vi "PlotData Loop.vi"(8 "error in":errorcluster, 9 "IBM OptoElectroMechanics Configuration":T1={"Parameter Analizer"={"Parameter Analyzer VISA Session"="COM1", "Sweeping Time Parameters"={"Integration Time"=0, "Short Integration Time (s)"=1.0, "Long Integration Time (s)"=0.0, "Wait Time Parameter"=1.0}, "Acquisition Mode"=enum."Sweeping Mode", "Status Polling Time (ms)"=0, "Comment"="Test VI", "SMU 1 - Sweeping"={"Start / Offset"=0.0, "Stop / Ratio"=1.0, "Step \n(linear only)"=0.01, "Compliance"=0.1, "Power \nCompliance"=0.0, "Mode"=0, "Function"=0, "Sweep Mode"=FALSE}, "SMU 2 - Sweeping"={"Start / Offset"=0.0, "Stop / Ratio"=1.0, "Step \n(linear only)"=0.01, "Compliance"=0.1, "Power \nCompliance"=0.0, "Mode"=0, "Function"=0, "Sweep Mode"=FALSE}, "SMU 3 - Sweeping"={"Start / Offset"=0.0, "Stop / Ratio"=1.0, "Step \n(linear only)"=0.01, "Compliance"=0.1, "Power \nCompliance"=0.0, "Mode"=0, "Function"=0, "Sweep Mode"=FALSE}, "SMU 4 - Sweeping"={"Start / Offset"=0.0, "Stop / Ratio"=1.0, "Step \n(linear only)"=0.01, "Compliance"=0.1, "Power \nCompliance"=0.0, "Mode"=0, "Function"=0, "Sweep Mode"=FALSE}, "Sweep Spacing"=0, "Range"=0, "SMU1 - Sampling"={"Source"=10.0, "Compliance"=1e-05, "Mode"=0, "Function"=FALSE}, "SMU2 - Sampling"={"Source"=1.0, "Compliance"=1.0, "Mode"=0, "Function"=FALSE}, "SMU3 - Sampling"={"Source"=10.0, "Compliance"=1e-05, "Mode"=0, "Function"=FALSE}, "SMU4 - Sampling"={"Source"=0.1, "Compliance"=60.0, "Mode"=10, "Function"=FALSE}, "Sampling Time Parameters"={"Initial Interval (s)"=0.1, "Number of Samples"=60, "Total Sampling Time (s)"=10.0, "Hold Time (s)"=0.0, "Sampling Mode"=0, "Sampling Time"=0}, "Stop Condition"={"Enable Delay (s)"=0.0, "Name"="", "Threshold"=0.0, "num. of events"=1, "Event"=0, "Stop Condition Enable"=FALSE}}, "Switching Matrix"={"Switching Matrix VISA Session"="GPIB0::18::INSTR", "Connections"=[{"Connections"=[FALSE, FALSE, FALSE, FALSE, FALSE, FALSE, FALSE, FALSE, FALSE, FALSE, FALSE, FALSE], "Connection Type"=enum."Disconnected"}, {"Connections"=[FALSE, FALSE, FALSE, FALSE, FALSE, FALSE, FALSE, FALSE, FALSE, FALSE, FALSE, FALSE], "Connection Type"=enum."Disconnected"}, {"Connections"=[FALSE, FALSE, FALSE, FALSE, FALSE, FALSE, FALSE, FALSE, FALSE, FALSE, FALSE, FALSE], "Connection Type"=enum."Disconnected"}, {"Connections"=[FALSE, FALSE, FALSE, FALSE, FALSE, FALSE, FALSE, FALSE, FALSE, FALSE, FALSE, FALSE], "Connection Type"=enum."Disconnected"}, {"Connections"=[FALSE, FALSE, FALSE, FALSE, FALSE, FALSE, FALSE, FALSE, FALSE, FALSE, FALSE, FALSE], "Connection Type"=enum."Disconnected"}, {"Connections"=[FALSE, FALSE, FALSE, FALSE, FALSE, FALSE, FALSE, FALSE, FALSE, FALSE, FALSE, FALSE], "Connection Type"=enum."Disconnected"}, {"Connections"=[FALSE, FALSE, FALSE, FALSE, FALSE, FALSE, FALSE, FALSE, FALSE, FALSE, FALSE, FALSE], "Connection Type"=enum."Disconnected"}, {"Connections"=[FALSE, FALSE, FALSE, FALSE, FALSE, FALSE, FALSE, FALSE, FALSE, FALSE, FALSE, FALSE], "Connection Type"=enum."Disconnected"}]}, "Stress Control"={"Stress Control VISA Session"="StrainMotor", "Axis"=0, "Motion"=0, "Destination (°)"=0.0, "Speed (°/s)"=4.0, "Position (°)"=25.0}, "Optical Spectrometer"={"Laser Settings"={"Laser Wavelength"=enum."365 nm", "Neutral Density Filter"=enum."100%"}, "Spectrometer Settings"={"Confocal Hole Size (µm)"=0.0, "Grating"=2, "Detector"=enum."InGaAs Array"}, "Acquisition Settings"={"Acquisition Mode"=enum."Multi-Window", "Spectal Position (nm)"=632.0, "From (nm)"=735.0, "To (nm)"=0.0, "Integration Time (s)"=0.0, "Number of Accumulations"=3, "AutoScanning"=FALSE, "Spike Removal"=FALSE}, "Path"=path "C:/07 - Prizes and Awards/Marie Curie Prize/Reply Editors Final NCOMMS(10).docx"}, "Switches & Mirrors"={"Relay VISA Session"="COM1", "Switches"={"Laser"=FALSE, "Video"=FALSE}, "Delays (ms)"={"Laser"=500, "Video"=1500}}, "Camera"={"Settings"={"Pixel clock"=20, "Frame rate"=30.0, "Exposure time"=33.21525, "Master Gain"=0, "Red Gain"=0, "Green Gain"=0, "Blue Gain"=0, "Auto Gain"=FALSE, "White-balance"=FALSE, "Color Correction"=FALSE}}, "XYZ Stage"={"Connection Settings"={"Tango VISA"="", "Baudrate"=57600, "Show Protocol?"=FALSE}, "Manual Control"={"North"=FALSE, "South"=FALSE, "West"=FALSE, "East"=FALSE, "Up"=FALSE, "Down"=FALSE, "Stop"=FALSE, "XY Step"=0.0, "Z step"=0.0}, "Coordinate Control"={"Motion Mode"=enum."Absolute", "Destination [mm]"=[]}}, "AutoFocus"={"Matching Criteria"={"Minimum Score"=700.0, "Color Score Weight"=700.0, "Minimum Contrast"=50, "Match Mode"=0, "Match Feature Mode"=0, "Subpixel Accuracy"=TRUE, "Color Sensitivity"=1, "Search Strategy"=1}, "Z Scan Parameters"={"Z Range"=1380.0, "Resolution"=5000.0, "Initial Direction"=enum."Up", "Focus Threshold"=0.1, "Ascent Constant"=0.1}, "Displacement"=0.0, "Transformation Matrix"=[]}, "Sava Data"={"Workspace Info"={"Device Name"="ProberHead_Tst_C29K3_7(2)", "Device Info"="ProberHead_Tst_C29", "Path"=path "C:/Users/gio/Desktop/ProbeHeadTest"}, "Instrument Configuration"={"Instrument"=enum."Unknown Instrument", "Configuration"="Test Configuration"}, "Stress Motor Position"=0.0, "Electrical Measurement"={"Sequence"=[], "V1"=[], "V2"=[], "V3"=[], "V4"=[], "I1"=[], "I2"=[], "I3"=[], "I4"=[]}, "Optical Spectrum"={"Intensity"=[], "Wavelength"=[], "Energy"=[], "Raman Shift"=[], "Detector Temperature"=0.0}}, "PlotData"={"Sliders"={"Strain Sequence"=0, "Instrument Sequence"=0}, "Measurement"={"Which Instrument?"=enum."No Plot", "Electrical Measurement"={"Sequence"=[], "V1"=[], "V2"=[], "V3"=[], "V4"=[], "I1"=[], "I2"=[], "I3"=[], "I4"=[]}, "Measurement Mode"=enum."Sweeping Mode", "Optical Spectrum"={"Intensity"=[], "Wavelength"=[], "Energy"=[], "Raman Shift"=[], "Detector Temperature"=0.0}}, "Instrument Steps"=[], "Strain Points"=[]}, "Instrument Sequence"={"Caller VI"=enum."User"}, "Strain Measurement"={"Stress Sequence "={"Max Motor Position"=1380.0, "# Intermediate Points"=5000, "Initial Direction"=enum."Tension"}, "Track?"=FALSE}} {"AutoFocus"."Displacement" scale=1.0..1000.0; "AutoFocus"."Z Scan Parameters"."Focus Threshold" min=0.0 max=1000.0 step=1.0 format="%#_2f"; "AutoFocus"."Z Scan Parameters"."Ascent Constant" min=0.0 max=1000.0 step=1.0 format="%#_2f"; "AutoFocus"."Z Scan Parameters"."Resolution" min=0.0 max=1.0 step=0.01 format="%_2g"; "AutoFocus"."Z Scan Parameters"."Z Range" format="%_3g"; "AutoFocus"."Matching Criteria"."Match Mode" items=["Shift Invariant", "Rotation Invariant"]; "AutoFocus"."Matching Criteria"."Match Feature Mode" items=["Color and Shape", "Color", "Shape"]; "AutoFocus"."Matching Criteria"."Color Sensitivity" items=["Low Sensitivity", "Medium Sensitivity", "High Sensitivity"]; "AutoFocus"."Matching Criteria"."Search Strategy" items=["Conservative", "Balance", "Aggressive", "Very Aggressive"]; "XYZ Stage"."Manual Control"."Z step" scale=0.1..10.0; "XYZ Stage"."Manual Control"."XY Step" scale=0.1..1000.0; "Camera"."Settings"."Blue Gain" min=0 max=100 scale=0.0..100.0; "Camera"."Settings"."Green Gain" min=0 max=100 scale=0.0..100.0; "Camera"."Settings"."Red Gain" min=0 max=100 scale=0.0..100.0; "Camera"."Settings"."Master Gain" min=0 max=100 scale=0.0..100.0; "Camera"."Settings"."Exposure time" min=0.101625 max=159.246375 step=0.101625 scale=0.101625..159.246375 scale format="%#.3g"; "Camera"."Settings"."Frame rate" min=2.7455631699174137 max=6.2675785993528725 step=0.000101625 scale=2.7455631699174137..6.2675785993528725 scale format="%^#_3g"; "Camera"."Settings"."Pixel clock" min=5 max=43 scale=5.0..43.0; "PlotData"."Sliders"."Instrument Sequence" scale=0.0..10.0; "PlotData"."Sliders"."Strain Sequence" scale=0.0..10.0; "Strain Measurement"."Stress Sequence"."# Intermediate Points" max=1390; "Parameter Analizer"."Stop Condition"."Event" items=["Value > Threshold", "Value < Threshold", "| Value | > | Threshold |", "| Value | < | Threshold |"]; "Parameter Analizer"."Stop Condition"."Threshold" format="%^.2e"; "Parameter Analizer"."Stop Condition"."Enable Delay (s)" format="%.1f"; "Parameter Analizer"."Sampling Time Parameters"."Sampling Time" items=["Auto (linear only)", "No Limit", "Set Limit"]; "Parameter Analizer"."Sampling Time Parameters"."Sampling Mode" items=["Linear", "Log10", "Log25", "Log50", "Thinned Out"]; "Parameter Analizer"."Sampling Time Parameters"."Hold Time (s)" format="%.4f"; "Parameter Analizer"."Sampling Time Parameters"."Total Sampling Time (s)" format="%.1f"; "Parameter Analizer"."Sampling Time Parameters"."Initial Interval (s)" format="%^.3e"; "Parameter Analizer"."SMU 4 - Sweeping"."Function" items=["Disabled", "Var 1", "Var 2", "Var 1'", "Constant"]; "Parameter Analizer"."SMU 4 - Sweeping"."Mode" items=["V", "I", "V pulse", "I  pulse", "Common"]; "Parameter Analizer"."SMU 4 - Sweeping"."Power \nCompliance" format="%^.2e"; "Parameter Analizer"."SMU 4 - Sweeping"."Compliance" format="%^.2e"; "Parameter Analizer"."SMU 4 - Sweeping"."Step \n(linear only)" format="%^.4e"; "Parameter Analizer"."SMU 4 - Sweeping"."Stop / Ratio" format="%^.4e"; "Parameter Analizer"."SMU 4 - Sweeping"."Start / Offset" format="%^.4e"; "Parameter Analizer"."SMU 3 - Sweeping"."Function" items=["Disabled", "Var 1", "Var 2", "Var 1'", "Constant"]; "Parameter Analizer"."SMU 3 - Sweeping"."Mode" items=["V", "I", "V pulse", "I  pulse", "Common"]; "Parameter Analizer"."SMU 3 - Sweeping"."Power \nCompliance" format="%^.2e"; "Parameter Analizer"."SMU 3 - Sweeping"."Compliance" format="%^.2e"; "Parameter Analizer"."SMU 3 - Sweeping"."Step \n(linear only)" format="%^.4e"; "Parameter Analizer"."SMU 3 - Sweeping"."Stop / Ratio" format="%^.4e"; "Parameter Analizer"."SMU 3 - Sweeping"."Start / Offset" format="%^.4e"; "Parameter Analizer"."SMU 2 - Sweeping"."Function" items=["Disabled", "Var 1", "Var 2", "Var 1'", "Constant"]; "Parameter Analizer"."SMU 2 - Sweeping"."Mode" items=["V", "I", "V pulse", "I  pulse", "Common"]; "Parameter Analizer"."SMU 2 - Sweeping"."Power \nCompliance" format="%^.2e"; "Parameter Analizer"."SMU 2 - Sweeping"."Compliance" format="%^.2e"; "Parameter Analizer"."SMU 2 - Sweeping"."Step \n(linear only)" format="%^.4e"; "Parameter Analizer"."SMU 2 - Sweeping"."Stop / Ratio" format="%^.4e"; "Parameter Analizer"."SMU 2 - Sweeping"."Start / Offset" format="%^.4e"; "Parameter Analizer"."SMU 1 - Sweeping"."Function" items=["Disabled", "Var 1", "Var 2", "Var 1'", "Constant"]; "Parameter Analizer"."SMU 1 - Sweeping"."Mode" items=["V", "I", "V pulse", "I  pulse", "Common"]; "Parameter Analizer"."SMU 1 - Sweeping"."Power \nCompliance" format="%^.2e"; "Parameter Analizer"."SMU 1 - Sweeping"."Compliance" format="%^.2e"; "Parameter Analizer"."SMU 1 - Sweeping"."Step \n(linear only)" format="%^.4e"; "Parameter Analizer"."SMU 1 - Sweeping"."Stop / Ratio" format="%^.4e"; "Parameter Analizer"."SMU 1 - Sweeping"."Start / Offset" format="%^.4e"; "Parameter Analizer"."Sweeping Time Parameters"."Long Integration Time (s)" scale=0.02..2.0; "Parameter Analizer"."Sweeping Time Parameters"."Short Integration Time (s)" scale=8e-05..0.00192; "Parameter Analizer"."Sweeping Time Parameters"."Integration Time" items=["Short", "Long"]; "Parameter Analizer"."Sweeping Time Parameters"."Wait Time Parameter" format="%.1f"; "Parameter Analizer"."SMU4 - Sampling"."Mode" items=["V", "I", "Common"]; "Parameter Analizer"."SMU4 - Sampling"."Compliance" format="%^.2e"; "Parameter Analizer"."SMU4 - Sampling"."Source" format="%^.3e"; "Parameter Analizer"."SMU3 - Sampling"."Mode" items=["V", "I", "Common"]; "Parameter Analizer"."SMU3 - Sampling"."Compliance" format="%^.2e"; "Parameter Analizer"."SMU3 - Sampling"."Source" format="%^.3e"; "Parameter Analizer"."SMU2 - Sampling"."Mode" items=["V", "I", "Common"]; "Parameter Analizer"."SMU2 - Sampling"."Compliance" format="%^.2e"; "Parameter Analizer"."SMU2 - Sampling"."Source" format="%^.3e"; "Parameter Analizer"."SMU1 - Sampling"."Mode" items=["V", "I", "Common"]; "Parameter Analizer"."SMU1 - Sampling"."Compliance" format="%^.2e"; "Parameter Analizer"."SMU1 - Sampling"."Source" format="%^.3e"; "Parameter Analizer"."Range" items=["auto", "fixed", "limited"]; "Parameter Analizer"."Sweep Spacing" items=["linear", "log 10", "log 25", "log 50"]; "Stress Control"."Axis" min=1 max=3; "Stress Control"."Position (°)" format="%.6g"; "Stress Control"."Speed (°/s)" min=0.0 max=4.0 format="%.6f"; "Stress Control"."Destination (°)" min=-2000000000.0 max=2000000000.0 format="%.6f"; "Stress Control"."Motion" items=["Absolute", "Relative"]; "Optical Spectrometer"."Spectrometer Settings"."Grating" items=["1800 l/mm", "150 l/mm"]}, 10 "Message Queues":T57, 11 "Notifiers":T44) -> (0 "error out":errorcluster)   [LabVIEW 2014]
uses:
  support/Message Queue/All Message Queues.ctl
  support/Message Queue/Message Cluster.ctl
  support/Notifiers/Notifiers.ctl
  support/Message Handler Loop Notifiers.ctl
  Hardware Control/Parameter Analyzer/Parameter Analyzer Notifiers.ctl
  Hardware Control/Switching Matrix/Switching Matrix Notifiers.ctl
  Hardware Control/Stress Control/StressControl Notifiers.ctl
  Hardware Control/Spectrometer/Spectrometer Notifiers.ctl
  Hardware Control/Switches and Mirrors/SwitchesMirrors Notifiers.ctl
  Hardware Control/Camera/Camera Notifiers.ctl
  Hardware Control/XYZ Stage/XYZ Notifications.ctl
  Hardware Control/Autofocus/Autofocus Notifiers.ctl
  Measurements/Optoelectronic Measurement/Optoelectronic Notifiers.ctl
  Measurements/Save Data/SaveData Notifiers.ctl
  Measurements/Instrument Sequence/Instrument Sequence Notifiers.ctl
  support/Configuration/Configuration.ctl
  Hardware Control/Parameter Analyzer/Parameter Analyzer Config.ctl
  Hardware Control/Parameter Analyzer/Parameter Analyzer Integration Parameters.ctl
  Hardware Control/Parameter Analyzer/Parameter Analyzer SMU Sweeping.ctl
  Hardware Control/Parameter Analyzer/Parameter Analyzer Sweep Spacing.ctl
  Hardware Control/Parameter Analyzer/Parameter Analyzer SMU Range.ctl
  Hardware Control/Parameter Analyzer/Parameter Analyzer SMU Sampling.ctl
  Hardware Control/Parameter Analyzer/Parameter Analyzer Sampling Parameters.ctl
  Hardware Control/Parameter Analyzer/Parameter Analyzer Stop Sampling Conditions.ctl
  Hardware Control/Switching Matrix/Switching Matrix Config.ctl
  Hardware Control/Stress Control/StressControl Config.ctl
  Hardware Control/Spectrometer/Spectrometer Config.ctl
  Hardware Control/Spectrometer/Laser Settings.ctl
  Hardware Control/Spectrometer/Laser.ctl
  Hardware Control/Spectrometer/Filter.ctl
  Hardware Control/Spectrometer/Grating Detector Settings.ctl
  Hardware Control/Spectrometer/Grating.ctl
  Hardware Control/Spectrometer/Detector.ctl
  Hardware Control/Spectrometer/Acquisition Settings.ctl
  Hardware Control/Switches and Mirrors/SwitchesMirrors Config.ctl
  Hardware Control/Switches and Mirrors/SwitchesMirrors Status.ctl
  Hardware Control/Camera/Camera Config.ctl
  Hardware Control/Camera/Camera Settings.ctl
  Hardware Control/XYZ Stage/XYZ Config.ctl
  Hardware Control/XYZ Stage/XYZ Connection Settings.ctl
  Hardware Control/XYZ Stage/XYZ Stage Control.ctl
  Hardware Control/XYZ Stage/XYZ Coordinate Control.ctl
  Hardware Control/Autofocus/AutoFocus Config.ctl
  Hardware Control/Autofocus/ZScan.ctl
  <vilib>/Analysis/Matrix/Datatypes/RealMatrix.ctl
  Measurements/Save Data/SaveData Config.ctl
  Measurements/Save Data/SaveData Workspace Info.ctl
  Measurements/Save Data/SaveData Instrument Configuration.ctl
  Measurements/Instrument Sequence/Instrument List.ctl
  Hardware Control/Spectrometer/Spectral Data.ctl
  Measurements/Plot Data/PlotData Config.ctl
  Measurements/Plot Data/Measurement.ctl
  Measurements/Plot Data/WhichInstrument.ctl
  Hardware Control/Parameter Analyzer/Electrical Data.ctl
  Measurements/Instrument Sequence/Instrument Steps.ctl
  Measurements/Instrument Sequence/Action.ctl
  Measurements/Instrument Sequence/Instrument Sequence Config.ctl
  Measurements/Strain Measurement/Strain Measurement Config.ctl
  Measurements/Plot Data/PlotData Functions.ctl
  support/Message Queue/Message Queue.lvlib
  <vilib>/Analysis/Matrix/NI_Matrix.lvlib
panel:
  # "LICENSED MATERIALS – PROPERTY OF IBM\nCopyright IBM Corp. 2016,\nALL RIGHTS RESERVED"
  # "XY"
  # "Z"
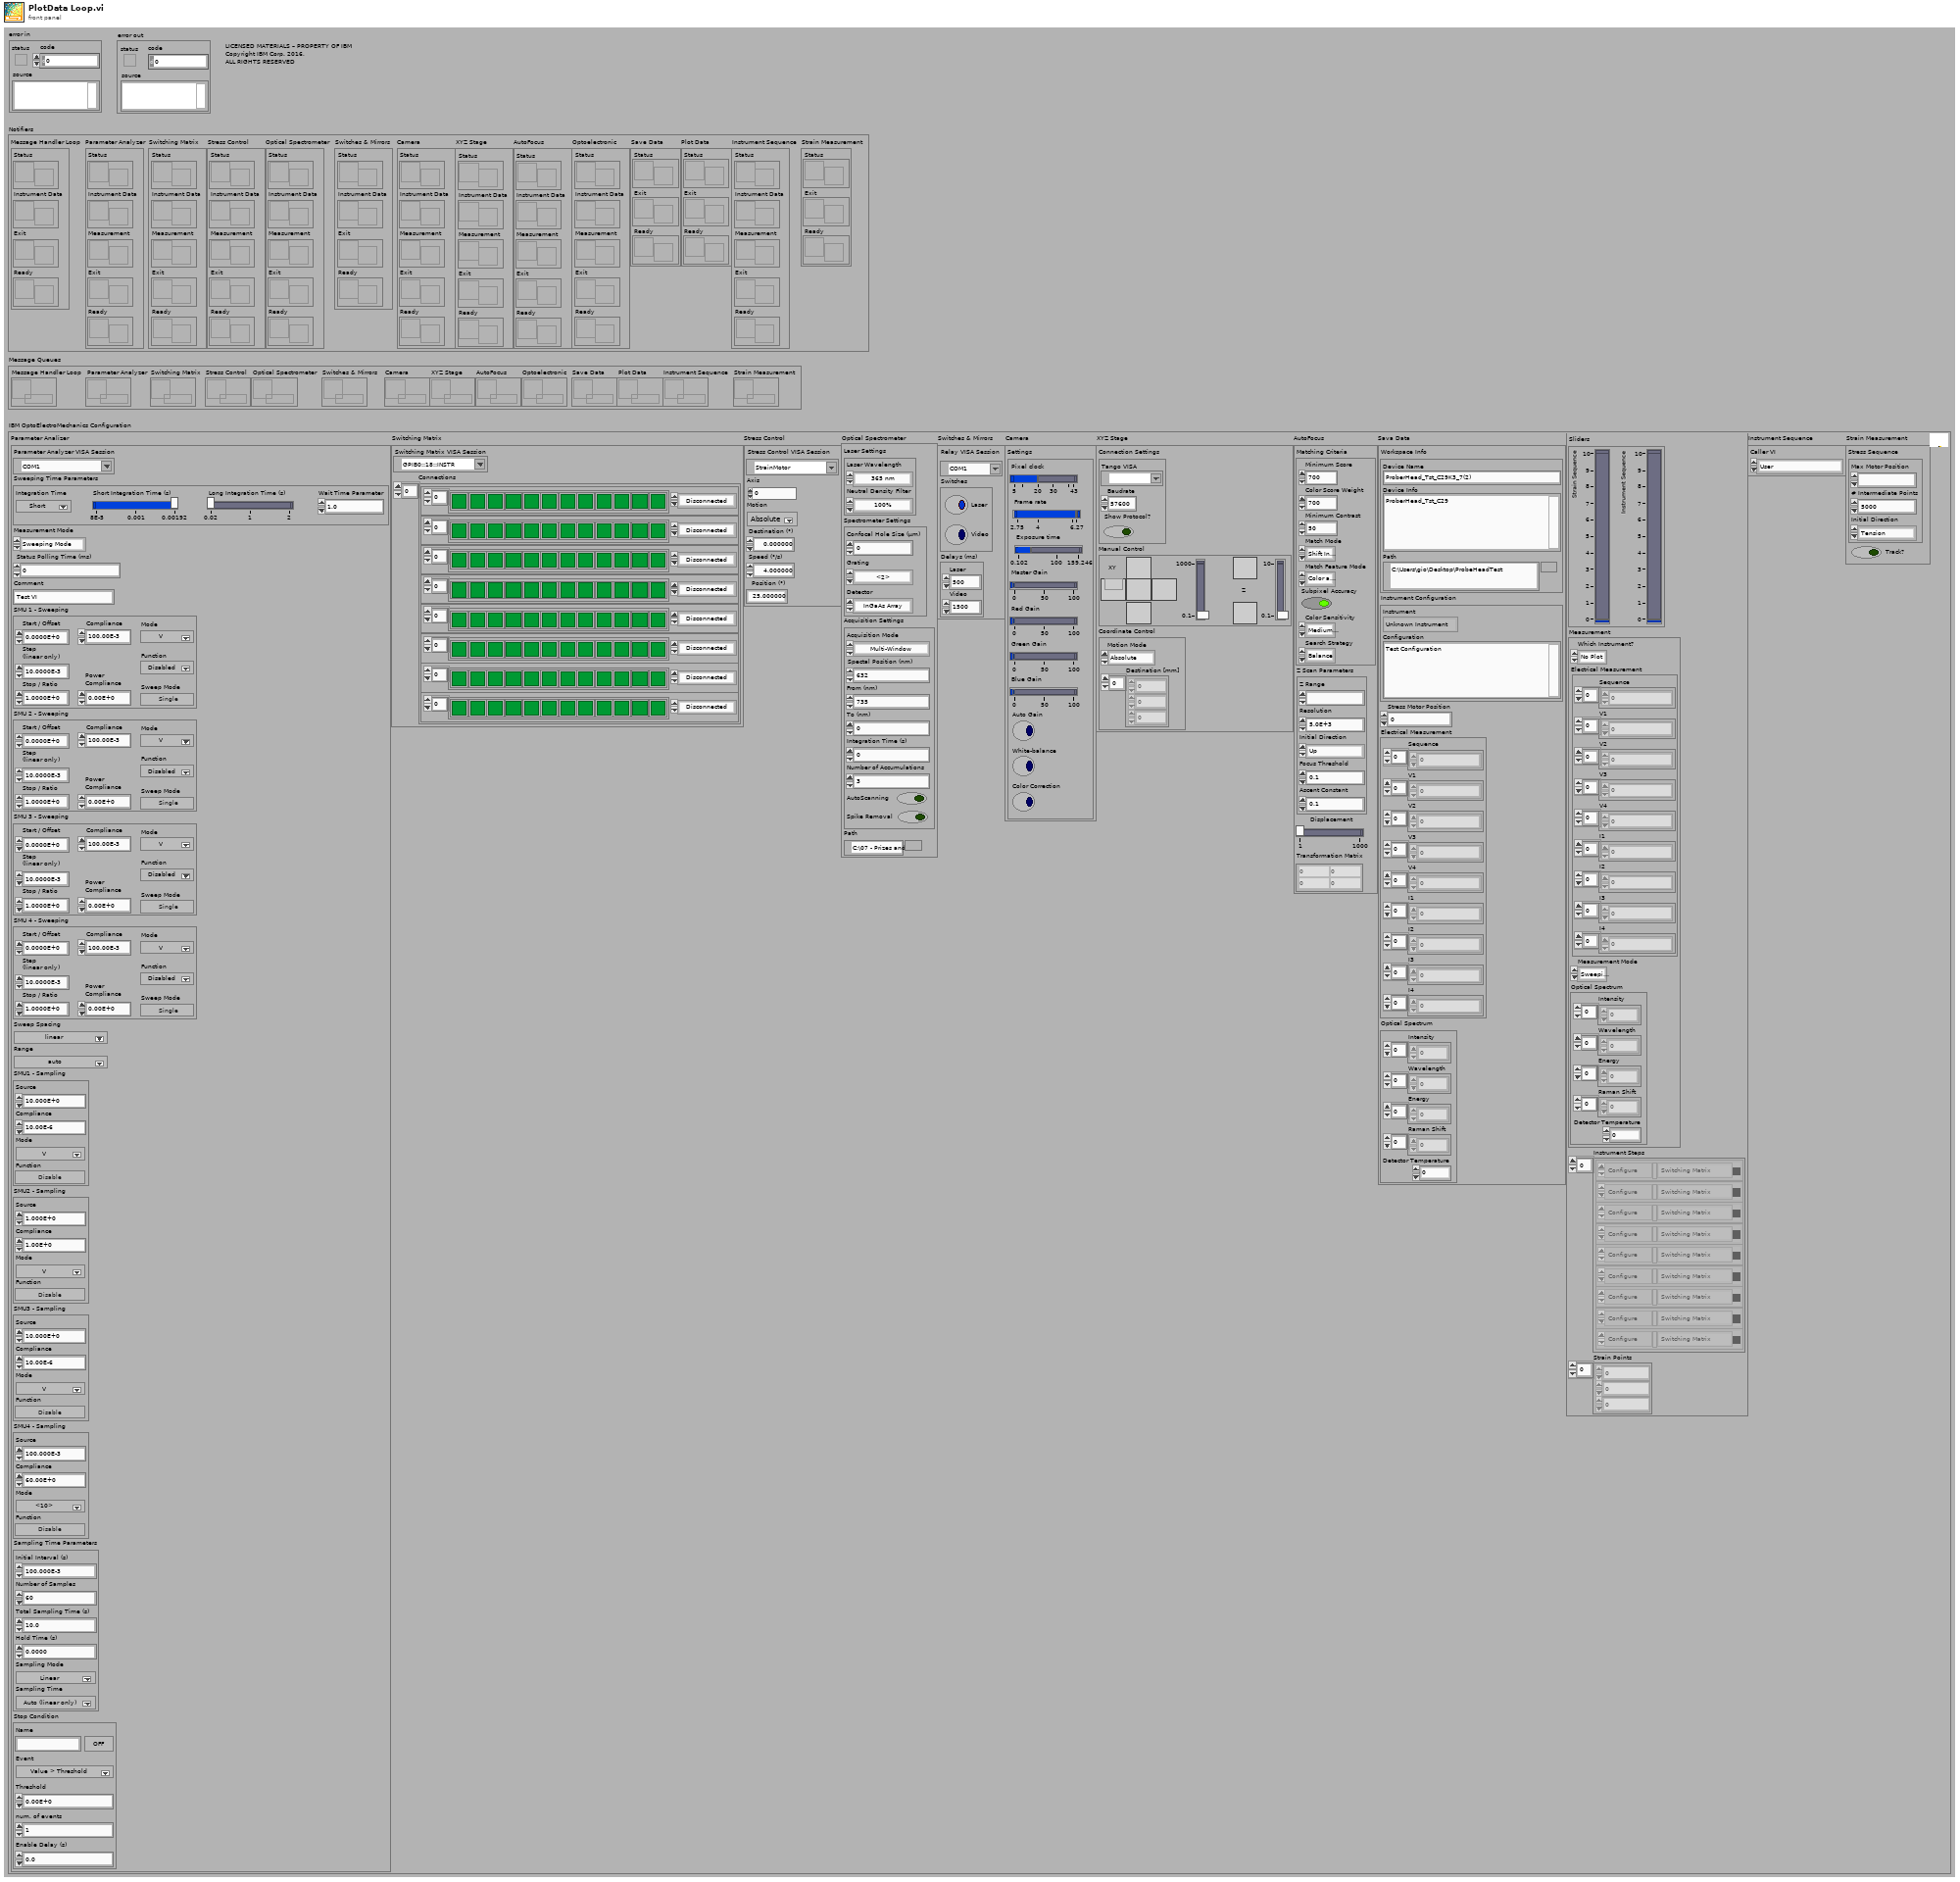
[diagram p1: front panel]
types:
  T1 = typedef "Configuration.ctl" = cluster{"Parameter Analizer":T2, "Switching Matrix":T10, "Stress Control":T11, "Optical Spectrometer":T12, "Switches & Mirrors":T20, "Camera":T22, "XYZ Stage":T24, "AutoFocus":T28, "Sava Data":T31, "PlotData":T36, "Instrument Sequence":T42, "Strain Measurement":T43}
  T2 = typedef "Parameter Analyzer Config.ctl" = cluster{"Parameter Analyzer VISA Session":refnum<visa-resource-name>, "Sweeping Time Parameters":T3, "Acquisition Mode":enum32{"Sweeping Mode", "Sampling Mode"}, "Status Polling Time (ms)":u32, "Comment":string, "SMU 1 - Sweeping":T4, "SMU 2 - Sweeping":T4, "SMU 3 - Sweeping":T4, "SMU 4 - Sweeping":T4, "Sweep Spacing":T5, "Range":T6, "SMU1 - Sampling":T7, "SMU2 - Sampling":T7, "SMU3 - Sampling":T7, "SMU4 - Sampling":T7, "Sampling Time Parameters":T8, "Stop Condition":T9}
  T3 = typedef "Parameter Analyzer Integration Parameters.ctl" = cluster{"Integration Time":u32, "Short Integration Time (s)":dbl, "Long Integration Time (s)":dbl, "Wait Time Parameter":dbl}
  T4 = typedef "Parameter Analyzer SMU Sweeping.ctl" = cluster{"Start / Offset":dbl, "Stop / Ratio":dbl, "Step \n(linear only)":dbl, "Compliance":dbl, "Power \nCompliance":dbl, "Mode":u32, "Function":i32, "Sweep Mode":bool}
  T5 = typedef "Parameter Analyzer Sweep Spacing.ctl" = u16
  T6 = typedef "Parameter Analyzer SMU Range.ctl" = u16
  T7 = typedef "Parameter Analyzer SMU Sampling.ctl" = cluster{"Source":dbl, "Compliance":dbl, "Mode":u32, "Function":bool}
  T8 = typedef "Parameter Analyzer Sampling Parameters.ctl" = cluster{"Initial Interval (s)":dbl, "Number of Samples":i32, "Total Sampling Time (s)":dbl, "Hold Time (s)":dbl, "Sampling Mode":i32, "Sampling Time":i32}
  T9 = typedef "Parameter Analyzer Stop Sampling Conditions.ctl" = cluster{"Enable Delay (s)":dbl, "Name":string, "Threshold":dbl, "num. of events":i32, "Event":i32, "Stop Condition Enable":bool}
  T10 = typedef "Switching Matrix Config.ctl" = cluster{"Switching Matrix VISA Session":refnum<visa-resource-name>, "Connections":cluster{"Connections":bool[], "Connection Type":enum16{"Disconnected", "Make - Break", "Break - Make"}}[]}
  T11 = typedef "StressControl Config.ctl" = cluster{"Stress Control VISA Session":refnum<visa-resource-name>, "Axis":i32, "Motion":u16, "Destination (°)":dbl, "Speed (°/s)":dbl, "Position (°)":dbl}
  T12 = typedef "Spectrometer Config.ctl" = cluster{"Laser Settings":T13, "Spectrometer Settings":T16, "Acquisition Settings":T19, "Path":path}
  T13 = typedef "Laser Settings.ctl" = cluster{"Laser Wavelength":T14, "Neutral Density Filter":T15}
  T14 = typedef "Laser.ctl" = enum16{"633 nm", "784 nm", "532 nm", "365 nm"}
  T15 = typedef "Filter.ctl" = enum16{"100%", "50%", "25%", "10%", "1%", "0.1%", "0.01%"}
  T16 = typedef "Grating Detector Settings.ctl" = cluster{"Confocal Hole Size (µm)":dbl, "Grating":T17, "Detector":T18}
  T17 = typedef "Grating.ctl" = u16
  T18 = typedef "Detector.ctl" = enum16{"InGaAs Array", "Silicon CCD"}
  T19 = typedef "Acquisition Settings.ctl" = cluster{"Acquisition Mode":enum16{"Single Window", "Multi-Window"}, "Spectal Position (nm)":dbl, "From (nm)":dbl, "To (nm)":dbl, "Integration Time (s)":dbl, "Number of Accumulations":i32, "AutoScanning":bool, "Spike Removal":bool}
  T20 = typedef "SwitchesMirrors Config.ctl" = cluster{"Relay VISA Session":refnum<visa-resource-name>, "Switches":T21, "Delays (ms)":cluster{"Laser":u32, "Video":u32}}
  T21 = typedef "SwitchesMirrors Status.ctl" = cluster{"Laser":bool, "Video":bool}
  T22 = typedef "Camera Config.ctl" = cluster{"Settings":T23}
  T23 = typedef "Camera Settings.ctl" = cluster{"Pixel clock":i32, "Frame rate":dbl, "Exposure time":dbl, "Master Gain":i32, "Red Gain":i32, "Green Gain":i32, "Blue Gain":i32, "Auto Gain":bool, "White-balance":bool, "Color Correction":bool}
  T24 = typedef "XYZ Config.ctl" = cluster{"Connection Settings":T25, "Manual Control":T26, "Coordinate Control":T27}
  T25 = typedef "XYZ Connection Settings.ctl" = cluster{"Tango VISA":refnum<visa-resource-name>, "Baudrate":i32, "Show Protocol?":bool}
  T26 = typedef "XYZ Stage Control.ctl" = cluster{"North":bool, "South":bool, "West":bool, "East":bool, "Up":bool, "Down":bool, "Stop":bool, "XY Step":dbl, "Z step":dbl}
  T27 = typedef "XYZ Coordinate Control.ctl" = cluster{"Motion Mode":enum16{"Absolute", "Relative"}, "Destination [mm]":dbl[]}
  T28 = typedef "AutoFocus Config.ctl" = cluster{"Matching Criteria":cluster{"Minimum Score":sgl, "Color Score Weight":sgl, "Minimum Contrast":i32, "Match Mode":u32, "Match Feature Mode":u32, "Subpixel Accuracy":bool, "Color Sensitivity":u32, "Search Strategy":u32}, "Z Scan Parameters":T29, "Displacement":dbl, "Transformation Matrix":T30}
  T29 = typedef "ZScan.ctl" = cluster{"Z Range":ext, "Resolution":dbl, "Initial Direction":enum16{"Up", "Down"}, "Focus Threshold":dbl, "Ascent Constant":dbl}
  T30 = typedef "NI_Matrix.lvlib/RealMatrix.ctl" = dbl[][]
  T31 = typedef "SaveData Config.ctl" = cluster{"Workspace Info":T32, "Instrument Configuration":T33, "Stress Motor Position":dbl, "Electrical Measurement":cluster{"Sequence":dbl[], "V1":dbl[], "V2":dbl[], "V3":dbl[], "V4":dbl[], "I1":dbl[], "I2":dbl[], "I3":dbl[], "I4":dbl[]}, "Optical Spectrum":T35}
  T32 = typedef "SaveData Workspace Info.ctl" = cluster{"Device Name":string, "Device Info":string, "Path":path}
  T33 = typedef "SaveData Instrument Configuration.ctl" = cluster{"Instrument":T34, "Configuration":string}
  T34 = typedef "Instrument List.ctl" = enum32{"Unknown Instrument", "Switching Matrix", "Parameter Analyzer", "Optical Spectrometer", "Optoelectronic", "Autofocus"}
  T35 = typedef "Spectral Data.ctl" = cluster{"Intensity":dbl[], "Wavelength":dbl[], "Energy":dbl[], "Raman Shift":dbl[], "Detector Temperature":dbl}
  T36 = typedef "PlotData Config.ctl" = cluster{"Sliders":cluster{"Strain Sequence":i32, "Instrument Sequence":i32}, "Measurement":T37, "Instrument Steps":T40, "Strain Points":dbl[]}
  T37 = typedef "Measurement.ctl" = cluster{"Which Instrument?":T38, "Electrical Measurement":T39, "Measurement Mode":enum16{"Sweeping Mode", "Sampling Mode"}, "Optical Spectrum":T35}
  T38 = typedef "WhichInstrument.ctl" = enum16{"No Plot", "Spectrometer", "Parameter Analyzer", "Optoelectronic"}
  T39 = typedef "Electrical Data.ctl" = cluster{"Sequence":dbl[], "V1":dbl[], "V2":dbl[], "V3":dbl[], "V4":dbl[], "I1":dbl[], "I2":dbl[], "I3":dbl[], "I4":dbl[]}
  T40 = typedef "Instrument Steps.ctl" = cluster{"Action":T41, "Configuration":variant, "Instrument":T34, "Status":enum8{"False", "True", "Mixed"}}[]
  T41 = typedef "Action.ctl" = enum32{"Configure", "Measure"}
  T42 = typedef "Instrument Sequence Config.ctl" = cluster{"Caller VI":enum16{"User", "Stress Measurement VI"}}
  T43 = typedef "Strain Measurement Config.ctl" = cluster{"Stress Sequence ":cluster{"Max Motor Position":ext, "# Intermediate Points":u32, "Initial Direction":enum16{"Tension", "Compression"}}, "Track?":bool}
  T44 = typedef "Notifiers.ctl" = cluster{"Message Handler Loop":T45, "Parameter Analyzer":T46, "Switching Matrix":T47, "Stress Control":T48, "Optical Spectrometer":T49, "Switches & Mirrors":T50, "Camera":T51, "XYZ Stage":T52, "AutoFocus":T53, "Optoelectronic":T54, "Save Data":T55, "Plot Data":T55, "Instrument Sequence":T56, "Strain Measurement":cluster{"Status":refnum<notifier>, "Exit":refnum<notifier>, "Ready":refnum<notifier>}}
  T45 = typedef "Message Handler Loop Notifiers.ctl" = cluster{"Status":refnum<notifier>, "Instrument Data":refnum<notifier>, "Exit":refnum<notifier>, "Ready":refnum<notifier>}
  T46 = typedef "Parameter Analyzer Notifiers.ctl" = cluster{"Status":refnum<notifier>, "Instrument Data":refnum<notifier>, "Measurement":refnum<notifier>, "Exit":refnum<notifier>, "Ready":refnum<notifier>}
  T47 = typedef "Switching Matrix Notifiers.ctl" = cluster{"Status":refnum<notifier>, "Instrument Data":refnum<notifier>, "Measurement":refnum<notifier>, "Exit":refnum<notifier>, "Ready":refnum<notifier>}
  T48 = typedef "StressControl Notifiers.ctl" = cluster{"Status":refnum<notifier>, "Instrument Data":refnum<notifier>, "Measurement":refnum<notifier>, "Exit":refnum<notifier>, "Ready":refnum<notifier>}
  T49 = typedef "Spectrometer Notifiers.ctl" = cluster{"Status":refnum<notifier>, "Instrument Data":refnum<notifier>, "Measurement":refnum<notifier>, "Exit":refnum<notifier>, "Ready":refnum<notifier>}
  T50 = typedef "SwitchesMirrors Notifiers.ctl" = cluster{"Status":refnum<notifier>, "Instrument Data":refnum<notifier>, "Exit":refnum<notifier>, "Ready":refnum<notifier>}
  T51 = typedef "Camera Notifiers.ctl" = cluster{"Status":refnum<notifier>, "Instrument Data":refnum<notifier>, "Measurement":refnum<notifier>, "Exit":refnum<notifier>, "Ready":refnum<notifier>}
  T52 = typedef "XYZ Notifications.ctl" = cluster{"Status":refnum<notifier>, "Instrument Data":refnum<notifier>, "Measurement":refnum<notifier>, "Exit":refnum<notifier>, "Ready":refnum<notifier>}
  T53 = typedef "Autofocus Notifiers.ctl" = cluster{"Status":refnum<notifier>, "Instrument Data":refnum<notifier>, "Measurement":refnum<notifier>, "Exit":refnum<notifier>, "Ready":refnum<notifier>}
  T54 = typedef "Optoelectronic Notifiers.ctl" = cluster{"Status":refnum<notifier>, "Instrument Data":refnum<notifier>, "Measurement":refnum<notifier>, "Exit":refnum<notifier>, "Ready":refnum<notifier>}
  T55 = typedef "SaveData Notifiers.ctl" = cluster{"Status":refnum<notifier>, "Exit":refnum<notifier>, "Ready":refnum<notifier>}
  T56 = typedef "Instrument Sequence Notifiers.ctl" = cluster{"Status":refnum<notifier>, "Instrument Data":refnum<notifier>, "Measurement":refnum<notifier>, "Exit":refnum<notifier>, "Ready":refnum<notifier>}
  T57 = typedef "Message Queue.lvlib/All Message Queues.ctl" = cluster{"Message Handler Loop":refnum<queue>, "Parameter Analyzer":refnum<queue>, "Switching Matrix":refnum<queue>, "Stress Control":refnum<queue>, "Optical Spectrometer":refnum<queue>, "Switches & Mirrors":refnum<queue>, "Camera":refnum<queue>, "XYZ Stage":refnum<queue>, "AutoFocus":refnum<queue>, "Optoelectronic":refnum<queue>, "Save Data":refnum<queue>, "Plot Data":refnum<queue>, "Instrument Sequence":refnum<queue>, "Strain Measurement":refnum<queue>}
  T58 = typedef "PlotData Data.ctl" = cluster{"Configuration":T36, "Refnums":T59, "Initialization":T62}
  T59 = typedef "PlotData Refnums.ctl" = cluster{"Choose Plot":refnum<vi>, "Instrument Sequence":refnum<vi>, "Strain Sequence":refnum<vi>, "Configuration":refnum<vi>, "Electrical Data Plot":T60, "Optical Spectrum Plot":T61, "Optoelectronic Plot":cluster{"Optical Spectrum Plot":T61, "Electrical Data Plot":T60}}
  T60 = typedef "Electrical Data Plot Refnums.ctl" = cluster{"Plot List":refnum<vi>, "Voltage Plot":refnum<vi>, "Current Plot":refnum<vi>, "IV Characteristic":refnum<vi>, "dI/dV-V Characteristic":refnum<vi>}
  T61 = typedef "Optical Spectrum Plot Refnum.ctl" = cluster{"Plot List":refnum<vi>, "Optical Spectrum vs Energy":refnum<vi>, "Optical Spectrum vs Wavelength":refnum<vi>, "Optical Spectrum vs Raman Shift":refnum<vi>, "Detector Temperature":refnum<vi>}
  T62 = typedef "PlotData Initialization.ctl" = cluster{"Update Refnums":bool}
  T63 = typedef "PlotData Functions.ctl" = enum16{"Set Config Array", "Set Strain Seq. Slider", "Desable Strain Seq. Slider", "Set Instrument Seq. Slider", "Desable Instrument Seq. Slider", "Clear Sequence", "Plot Data", "Append Measurement", "Next Strain Step", "Update Refnums"}
  T64 = cluster{"Strain Sequence":i32, "Instrument Sequence":i32}
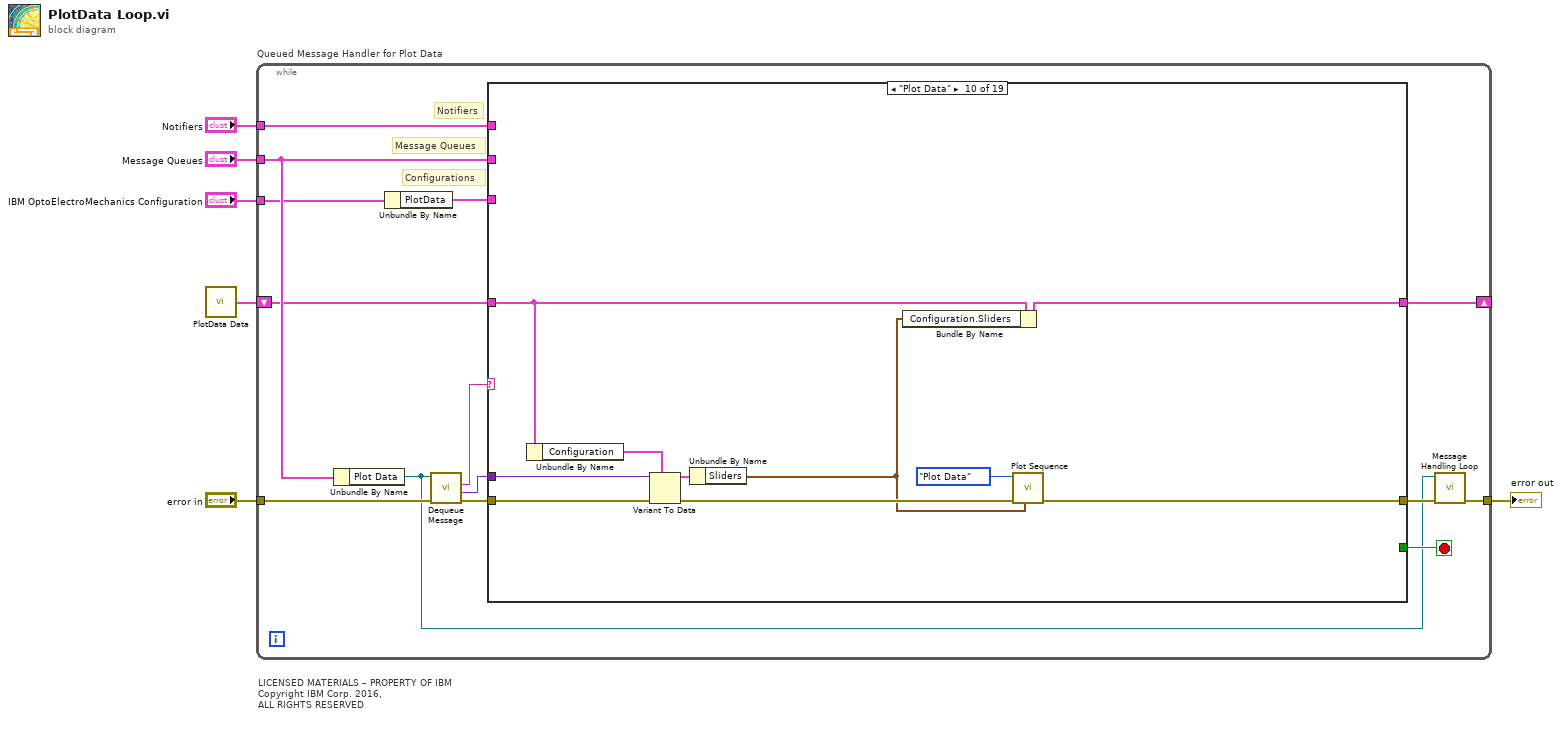
[diagram p0: block diagram]
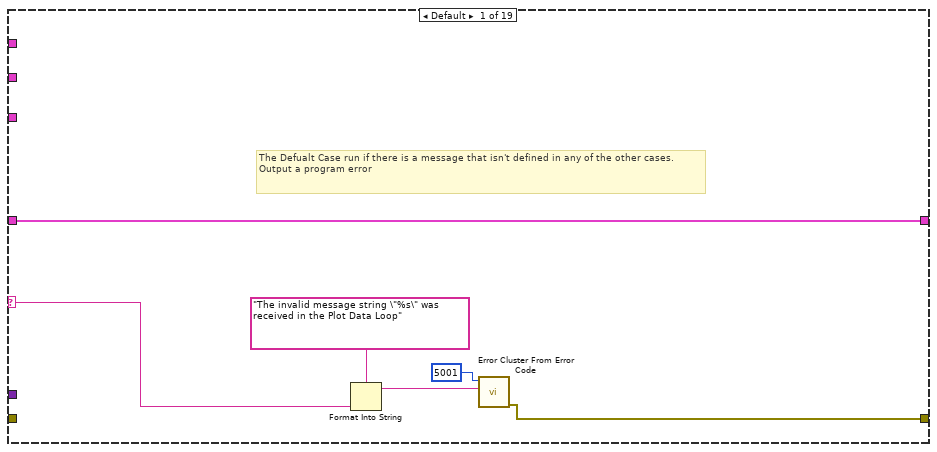
[diagram p2: hidden frame]
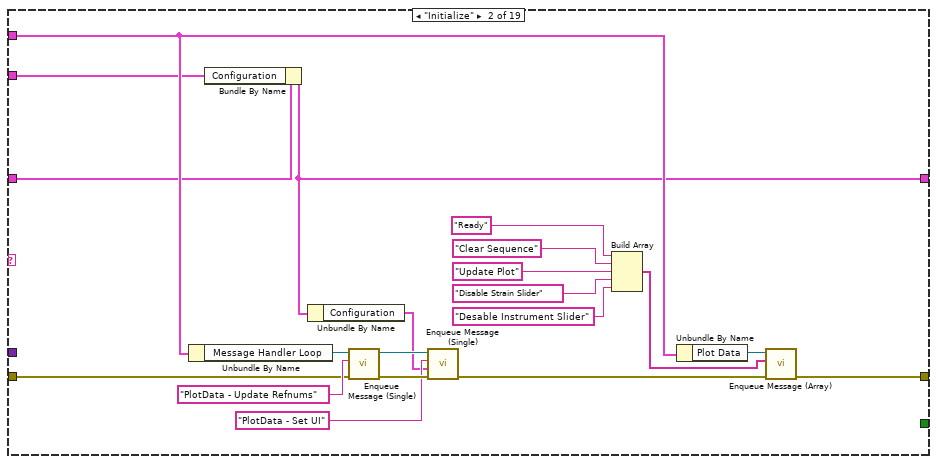
[diagram p3: hidden frame]
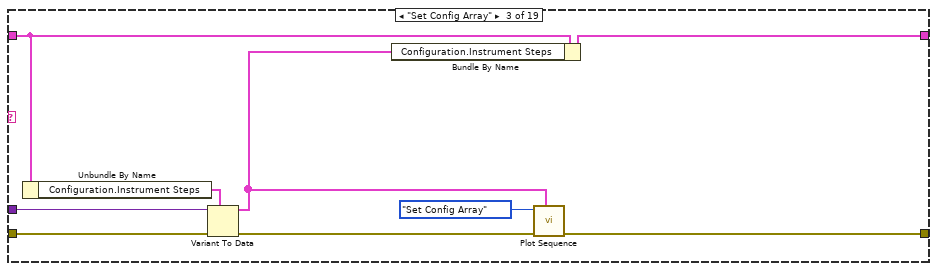
[diagram p4: hidden frame]
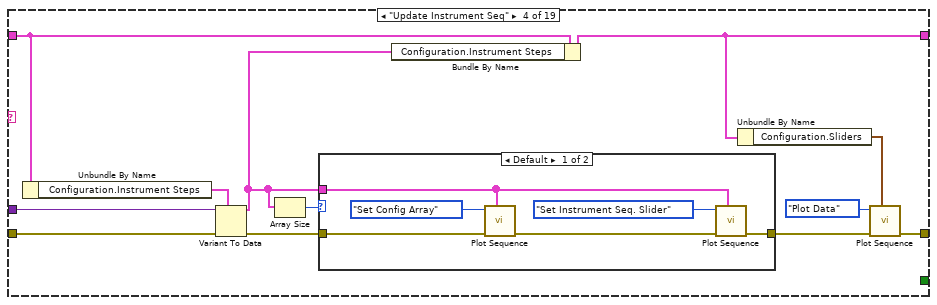
[diagram p5: hidden frame]
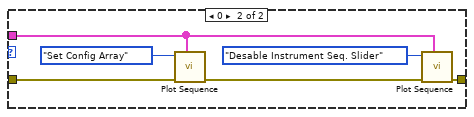
[diagram p6: hidden frame]
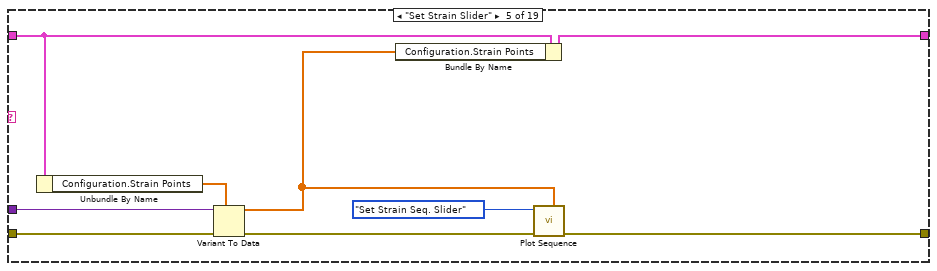
[diagram p7: hidden frame]
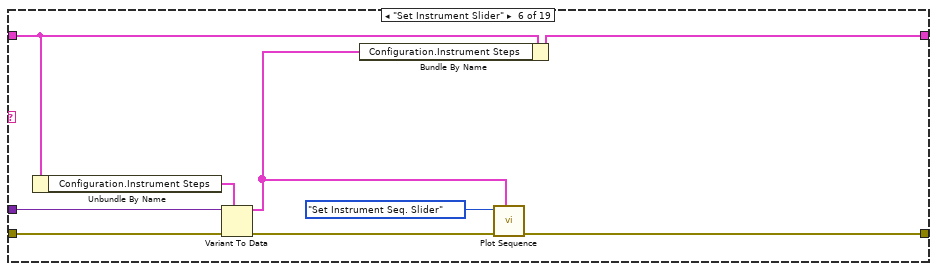
[diagram p8: hidden frame]
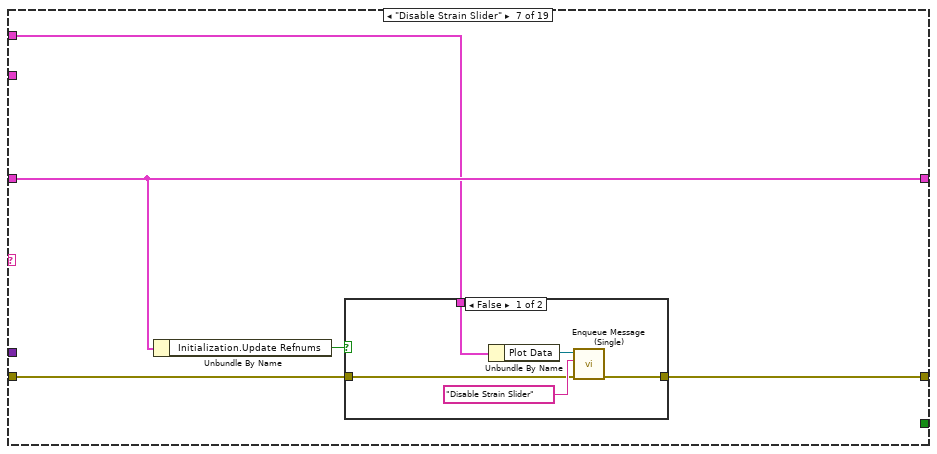
[diagram p9: hidden frame]
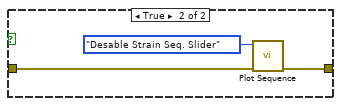
[diagram p10: hidden frame]
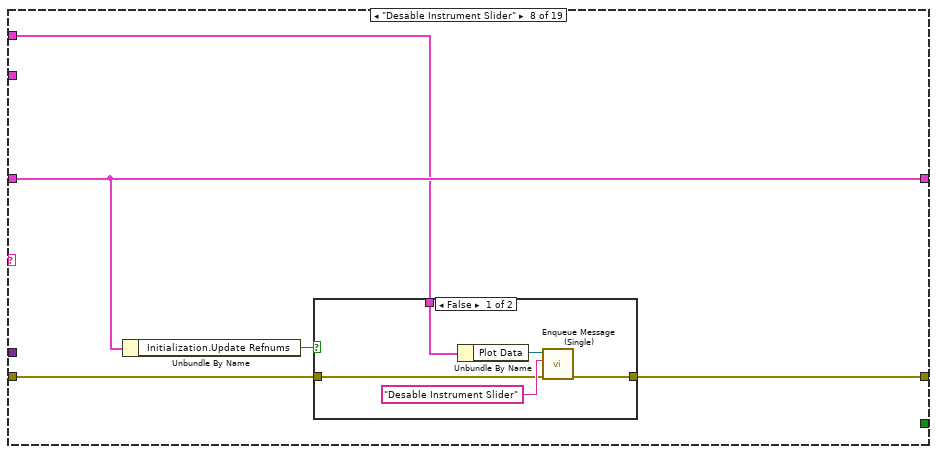
[diagram p11: hidden frame]
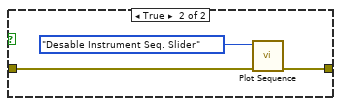
[diagram p12: hidden frame]
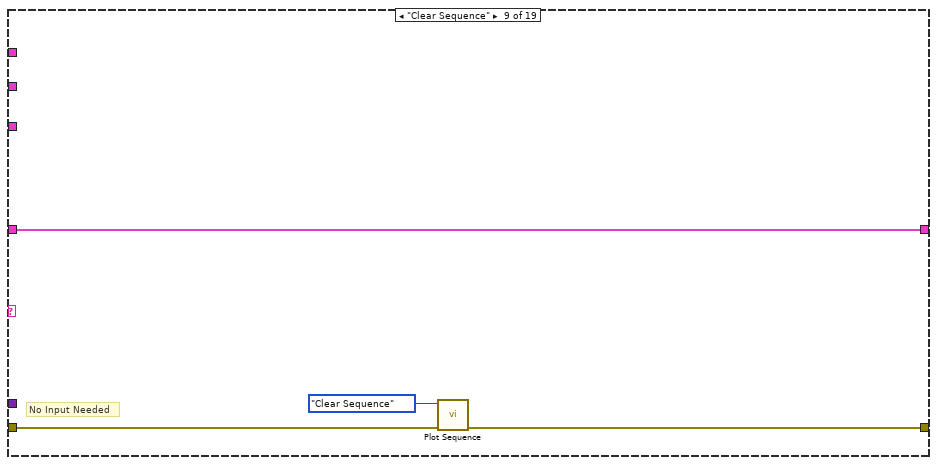
[diagram p13: hidden frame]
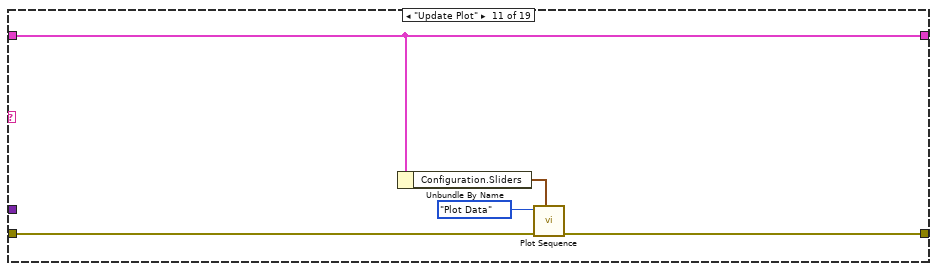
[diagram p14: hidden frame]
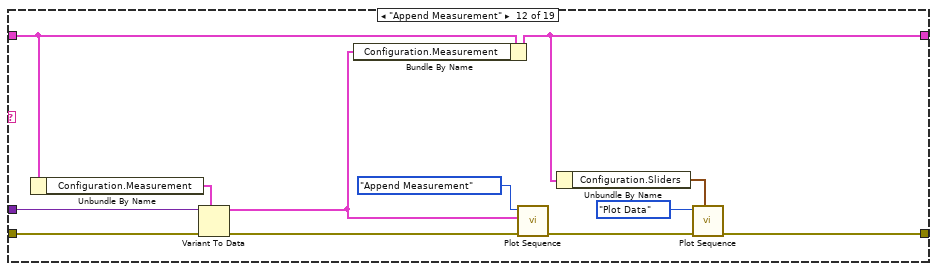
[diagram p15: hidden frame]
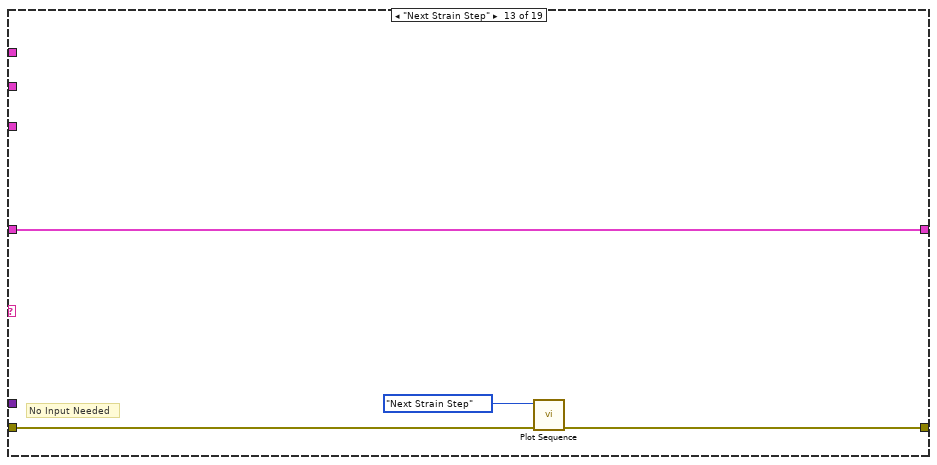
[diagram p16: hidden frame]
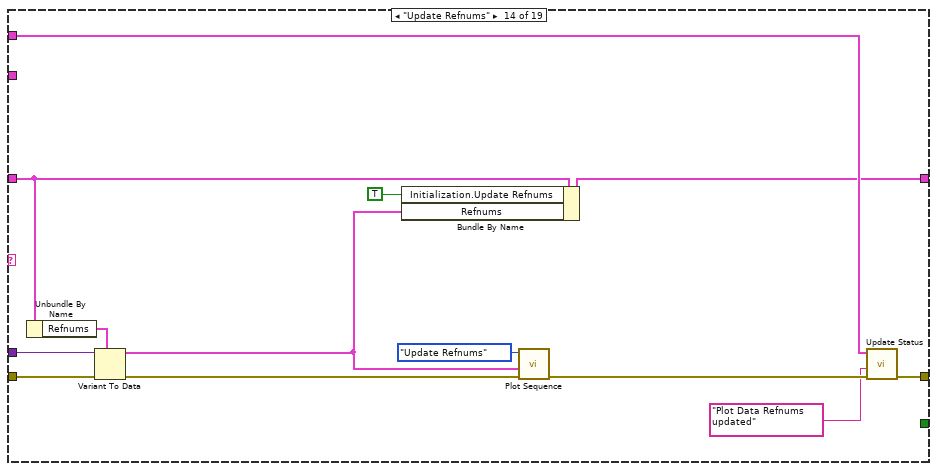
[diagram p17: hidden frame]
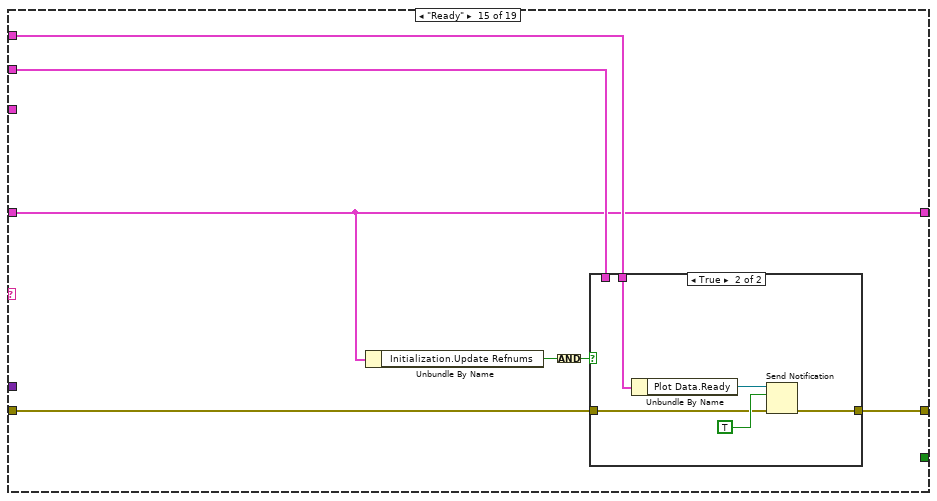
[diagram p18: hidden frame]
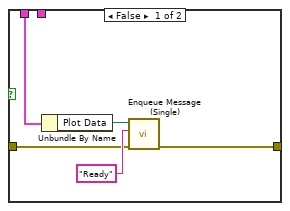
[diagram p19: hidden frame]
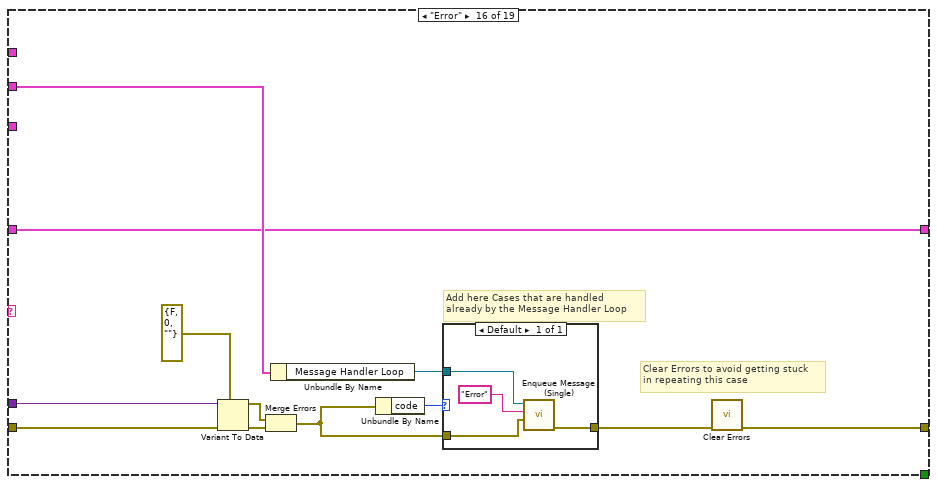
[diagram p20: hidden frame]
diagram:
  # "LICENSED MATERIALS – PROPERTY OF IBM\nCopyright IBM Corp. 2016,\nALL RIGHTS RESERVED"
  n1 = call "PlotData Data.vi"() -> ("Plot Data"=w2:T58)
  n2 = while "Queued Message Handler for Plot Data" {
    tunnel: "error in" -> [w20]
    tunnel: [w12] -> w3
    tunnel: "Message Queues" -> [w16]
    tunnel: "Notifiers" -> [w15]
    shift-right: [w10] -> _
    shift-left: w2 -> [w9]
    tunnel: "IBM OptoElectroMechanics Configuration" -> [w8]
    stop <- w14 stop-if-true
    # "Configurations"
    # "Notifiers"
    # "Message Queues"
    n3 = Unbundle By Name(w16) -> ("Plot Data"=w11:refnum<queue>)
    n4 = Unbundle By Name(w8) -> ("PlotData"=w7:T36)
    n5 = call "Dequeue Message.vi"("error in (no error)"=w20, "Message Queue"=w11) -> ("error out"=w19:errorcluster, "Message Data"=w17:variant, "Message"=w18:string)  [unwired: 7 out]
    n6 = case shown="\"Plot Data\"" w18 {
      selector: w18 -> [w23 _ _ _ _ _ _ _ _ _ _ _ _ _ _ _ _ _ _]
      tunnel: w19 -> [_ w43 w53 w67 w87 w96 w101 w114 w127 w136 w138 w154 w157 w171 w178 w197 w212 w220 w234]
      tunnel: [w22 w33 w55 w57 w88 w97 w100 w115 w124 w137 w142 w143 w158 w164 w176 w192 w205 w219 w236] -> w13
      tunnel: w17 -> [_ _ w51 w65 w84 w93 _ _ _ w133 _ w151 _ w168 _ w190 _ _ _]
      tunnel: w16 -> [_ w42 _ _ _ _ w98 w111 _ _ _ _ _ w163 w177 w198 w215 w218 w235]
      tunnel: w15 -> [_ _ _ _ _ _ _ _ _ _ _ _ _ _ w175 _ w207 _ _]
      tunnel: [_ _ _ _ _ _ _ _ _ _ _ _ _ _ _ _ TRUE ("Priority Message? (F)") _ _] -> w14
      tunnel: [w21 w35 w48 w56 w81 w90 w99 w113 w125 w130 w140 w144 w155 w161 w173 w189 w213 w217 w233] -> w10
      tunnel: w9 -> [w21 w37 w50 w64 w83 w92 w99 w113 w125 w132 w140 w150 w155 w167 w173 w189 w213 w217 w233]
      tunnel: w7 -> [_ w36 _ _ _ _ _ _ _ _ _ _ _ _ _ _ _ _ _]
      frame Default {
        # "The Defualt Case run if there is a message that isn't defined in any of the other cases.\nOutput a program error"
        n7 = Format Into String(format string="The invalid message string \"%s\" was  received in the Plot Data Loop", w23) -> (resulting string=w25:string)  [unwired: 2 in, 1 out]
        n8 = call <vilib>:"Error Cluster From Error Code.vi"("error message (\"\")"=w25, "error code (0)"=5001) -> ("error out"=w22:errorcluster)  [unwired: 2 in, 5 out]
      }
      frame "Initialize" {
        n9 = Unbundle By Name(w42) -> ("Message Handler Loop"=w45:refnum<queue>)
        n10 = Bundle By Name(cluster=w37, "Configuration"=w36) -> (w35:T58)
        n11 = Unbundle By Name(w35) -> ("Configuration"=w34:T36)
        n12 = call "Enqueue Message (Single).vi"("error in (no error)"=w43, "Message"="PlotData - Update Refnums", "Message Queue"=w45) -> ("error out"=w41:errorcluster, "dup Message Queue"=w40:refnum<queue>)  [unwired: 1 in, 6 out]
        n13 = call "Enqueue Message (Single).vi"("error in (no error)"=w41, "Message Data"=w34, "Message"="PlotData - Set UI", "Message Queue"=w40) -> ("error out"=w39:errorcluster)  [unwired: 7 out]
        n14 = Build Array("Ready" ("Message"), "Clear Sequence" ("Message"), "Update Plot" ("Message"), "Disable Strain Slider" ("Message"), "Desable Instrument Slider" ("Message")) -> (w32:string[])
        n15 = Unbundle By Name(w42) -> ("Plot Data"=w46:refnum<queue>)
        n16 = call "Enqueue Message (Array).vi"("error in (no error)"=w39, "Message Array"=w32, "Message Queue"=w46) -> ("error out"=w33:errorcluster)  [unwired: 1 in, 7 out]
      }
      frame "Set Config Array" {
        n17 = Unbundle By Name(w50) -> ("Configuration.Instrument Steps"=w49:T40)
        n18 = Variant To Data(error in=w53, type=w49, Variant=w51) -> (data=w47:T40, error out=w52:errorcluster)
        n19 = Bundle By Name(cluster=w50, "Configuration.Instrument Steps"=w47) -> (w48:T58)
        n20 = call "Plot Sequence.vi"("Instrument Steps"=w47, "error in (no error)"=w52, "Function"=PlotData_Functions."Set Config Array") -> ("error out"=w55:errorcluster)  [unwired: 4 in, 4 out]
      }
      frame "Update Instrument Seq" {
        n21 = Unbundle By Name(w64) -> ("Configuration.Instrument Steps"=w63:T40)
        n22 = Variant To Data(error in=w67, type=w63, Variant=w65) -> (data=w61:T40, error out=w66:errorcluster)
        n23 = Array Size(array=w61) -> (size(s)=w62:i32)
        n24 = case shown="Default" w62 {
          tunnel: w66 -> [w72 w78]
          tunnel: [w70 w76] -> w58
          tunnel: w61 -> [w69 w75]
          frame Default {
            n25 = call "Plot Sequence.vi"("Instrument Steps"=w69, "error in (no error)"=w72, "Function"=PlotData_Functions."Set Config Array") -> ("error out"=w71:errorcluster)  [unwired: 4 in, 4 out]
            n26 = call "Plot Sequence.vi"("Instrument Steps"=w69, "error in (no error)"=w71, "Function"=PlotData_Functions."Set Instrument Seq. Slider") -> ("error out"=w70:errorcluster)  [unwired: 4 in, 4 out]
          }
          frame 0 {
            n27 = call "Plot Sequence.vi"("Instrument Steps"=w75, "error in (no error)"=w78, "Function"=PlotData_Functions."Set Config Array") -> ("error out"=w77:errorcluster)  [unwired: 4 in, 4 out]
            n28 = call "Plot Sequence.vi"("Instrument Steps"=w75, "error in (no error)"=w77, "Function"=PlotData_Functions."Desable Instrument Seq. Slider") -> ("error out"=w76:errorcluster)  [unwired: 4 in, 4 out]
          }
        }
        n29 = Bundle By Name(cluster=w64, "Configuration.Instrument Steps"=w61) -> (w56:T58)
        n30 = Unbundle By Name(w56) -> ("Configuration.Sliders"=w60:T64)
        n31 = call "Plot Sequence.vi"("Sliders"=w60, "error in (no error)"=w58, "Function"=PlotData_Functions."Plot Data") -> ("error out"=w57:errorcluster)  [unwired: 4 in, 4 out]
      }
      frame "Set Strain Slider" {
        n32 = Unbundle By Name(w83) -> ("Configuration.Strain Points"=w82:dbl[])
        n33 = Variant To Data(error in=w87, type=w82, Variant=w84) -> (data=w80:dbl[], error out=w85:errorcluster)
        n34 = Bundle By Name(cluster=w83, "Configuration.Strain Points"=w80) -> (w81:T58)
        n35 = call "Plot Sequence.vi"("Strain Points"=w80, "error in (no error)"=w85, "Function"=PlotData_Functions."Set Strain Seq. Slider") -> ("error out"=w88:errorcluster)  [unwired: 4 in, 4 out]
      }
      frame "Set Instrument Slider" {
        n36 = Unbundle By Name(w92) -> ("Configuration.Instrument Steps"=w91:T40)
        n37 = Variant To Data(error in=w96, type=w91, Variant=w93) -> (data=w89:T40, error out=w94:errorcluster)
        n38 = Bundle By Name(cluster=w92, "Configuration.Instrument Steps"=w89) -> (w90:T58)
        n39 = call "Plot Sequence.vi"("Instrument Steps"=w89, "error in (no error)"=w94, "Function"=PlotData_Functions."Set Instrument Seq. Slider") -> ("error out"=w97:errorcluster)  [unwired: 4 in, 4 out]
      }
      frame "Disable Strain Slider" {
        n40 = Unbundle By Name(w99) -> ("Initialization.Update Refnums"=w102:bool)
        n41 = case shown="False" w102 {
          tunnel: [w105 w110] -> w100
          tunnel: w101 -> [w104 w108]
          tunnel: w98 -> [w103 _]
          frame False {
            n42 = Unbundle By Name(w103) -> ("Plot Data"=w106:refnum<queue>)
            n43 = call "Enqueue Message (Single).vi"("error in (no error)"=w104, "Message"="Disable Strain Slider", "Message Queue"=w106) -> ("error out"=w105:errorcluster)  [unwired: 1 in, 7 out]
          }
          frame True {
            n44 = call "Plot Sequence.vi"("error in (no error)"=w108, "Function"=PlotData_Functions."Desable Strain Seq. Slider") -> ("error out"=w110:errorcluster)  [unwired: 5 in, 4 out]
          }
        }
      }
      frame "Desable Instrument Slider" {
        n45 = Unbundle By Name(w113) -> ("Initialization.Update Refnums"=w112:bool)
        n46 = case shown="False" w112 {
          tunnel: [w118 w123] -> w115
          tunnel: w114 -> [w117 w121]
          tunnel: w111 -> [w116 _]
          frame False {
            n47 = Unbundle By Name(w116) -> ("Plot Data"=w119:refnum<queue>)
            n48 = call "Enqueue Message (Single).vi"("error in (no error)"=w117, "Message"="Desable Instrument Slider", "Message Queue"=w119) -> ("error out"=w118:errorcluster)  [unwired: 1 in, 7 out]
          }
          frame True {
            n49 = call "Plot Sequence.vi"("error in (no error)"=w121, "Function"=PlotData_Functions."Desable Instrument Seq. Slider") -> ("error out"=w123:errorcluster)  [unwired: 5 in, 4 out]
          }
        }
      }
      frame "Clear Sequence" {
        # "No Input Needed"
        n50 = call "Plot Sequence.vi"("error in (no error)"=w127, "Function"=PlotData_Functions."Clear Sequence") -> ("error out"=w124:errorcluster)  [unwired: 5 in, 4 out]
      }
      frame "Plot Data" {
        n51 = Unbundle By Name(w132) -> ("Configuration"=w131:T36)
        n52 = Variant To Data(error in=w136, type=w131, Variant=w133) -> (data=w129:T36, error out=w134:errorcluster)
        n53 = Unbundle By Name(w129) -> ("Sliders"=w128:T64)
        n54 = Bundle By Name(cluster=w132, "Configuration.Sliders"=w128) -> (w130:T58)
        n55 = call "Plot Sequence.vi"("Sliders"=w128, "error in (no error)"=w134, "Function"=PlotData_Functions."Plot Data") -> ("error out"=w137:errorcluster)  [unwired: 4 in, 4 out]
      }
      frame "Update Plot" {
        n56 = Unbundle By Name(w140) -> ("Configuration.Sliders"=w139:T64)
        n57 = call "Plot Sequence.vi"("Sliders"=w139, "error in (no error)"=w138, "Function"=PlotData_Functions."Plot Data") -> ("error out"=w142:errorcluster)  [unwired: 4 in, 4 out]
      }
      frame "Append Measurement" {
        n58 = Unbundle By Name(w150) -> ("Configuration.Measurement"=w149:T37)
        n59 = Variant To Data(error in=w154, type=w149, Variant=w151) -> (data=w148:T37, error out=w152:errorcluster)
        n60 = Bundle By Name(cluster=w150, "Configuration.Measurement"=w148) -> (w144:T58)
        n61 = call "Plot Sequence.vi"("error in (no error)"=w152, "Measurement"=w148, "Function"=PlotData_Functions."Append Measurement") -> ("error out"=w145:errorcluster)  [unwired: 4 in, 4 out]
        n62 = Unbundle By Name(w144) -> ("Configuration.Sliders"=w147:T64)
        n63 = call "Plot Sequence.vi"("Sliders"=w147, "error in (no error)"=w145, "Function"=PlotData_Functions."Plot Data") -> ("error out"=w143:errorcluster)  [unwired: 4 in, 4 out]
      }
      frame "Next Strain Step" {
        # "No Input Needed"
        n64 = call "Plot Sequence.vi"("error in (no error)"=w157, "Function"=PlotData_Functions."Next Strain Step") -> ("error out"=w158:errorcluster)  [unwired: 5 in, 4 out]
      }
      frame "Update Refnums" {
        n65 = Unbundle By Name(w167) -> ("Refnums"=w166:T59)
        n66 = Variant To Data(error in=w171, type=w166, Variant=w168) -> (data=w159:T59, error out=w169:errorcluster)
        n67 = Bundle By Name(cluster=w167, "Initialization.Update Refnums"=TRUE, "Refnums"=w159) -> (w161:T58)
        n68 = call "Plot Sequence.vi"("error in (no error)"=w169, "Refnums"=w159, "Function"=PlotData_Functions."Update Refnums") -> ("error out"=w165:errorcluster)  [unwired: 4 in, 4 out]
        n69 = call "Update Status.vi"("error in"=w165, "String"="Plot Data Refnums updated" ("button name (\"OK\")"), "Message Queues out"=w163) -> ("error out"=w164:errorcluster)  [unwired: 8 out]
      }
      frame "Ready" {
        n70 = Unbundle By Name(w173) -> ("Initialization.Update Refnums"=w172:bool)
        n71 = Compound Arithmetic op=AND(w172) -> (w174:bool)
        n72 = case shown="True" w174 {
          tunnel: [w181 w186] -> w176
          tunnel: w178 -> [w180 w185]
          tunnel: w177 -> [w179 _]
          tunnel: w175 -> [_ w184]
          frame False {
            n73 = Unbundle By Name(w179) -> ("Plot Data"=w183:refnum<queue>)
            n74 = call "Enqueue Message (Single).vi"("error in (no error)"=w180, "Message"="Ready", "Message Queue"=w183) -> ("error out"=w181:errorcluster)  [unwired: 1 in, 7 out]
          }
          frame True {
            n75 = Unbundle By Name(w184) -> ("Plot Data.Ready"=w187:refnum<notifier>)
            n76 = Send Notification(notification=TRUE, notifier=w187, error in (no error)=w185) -> (error out=w186:errorcluster)  [unwired: 1 out]
          }
        }
      }
      frame "Error" {
        # "Clear Errors to avoid getting stuck \nin repeating this case"
        # "Add here Cases that are handled \nalready by the Message Handler Loop"
        n77 = Variant To Data(error in=w197, type=errorcluster {"status"=FALSE, "code"=0, "source"=""} ("error out"), Variant=w190) -> (data=w196:errorcluster, error out=w195:errorcluster)
        n78 = Merge Errors(w196, w195) -> (w194:errorcluster)
        n79 = Unbundle By Name(w198) -> ("Message Handler Loop"=w200:refnum<queue>)
        n80 = Unbundle By Name(w194) -> ("code"=w191:i32)
        n81 = case shown="Default" w191 {
          tunnel: w200 -> [w204]
          tunnel: w194 -> [w202]
          tunnel: [w201] -> w193
          frame Default {
            n82 = call "Enqueue Message (Single).vi"("Message Data"=w202, "Message"="Error", "Message Queue"=w204) -> ("error out"=w201:errorcluster)  [unwired: 1 in, 7 out]
          }
        }
        n83 = call <vilib>:"Clear Errors.vi"("error in (no error)"=w193) -> ("error out"=w192:errorcluster)  [unwired: 1 in, 5 out]
      }
      frame "Exit" {
        w210 = TRUE ("Priority Message? (F)")
        # "Stop the VI"
        n84 = Unbundle By Name(w215) -> ("Plot Data"=w216:refnum<queue>)
        n85 = Release Queue(queue=w216, error in (no error)=w212) -> (error out=w206:errorcluster)  [unwired: 3 out]
        n86 = Unbundle By Name(w207) -> ("Plot Data.Exit"=w211:refnum<notifier>, "Plot Data.Ready"=w208:refnum<notifier>)
        n87 = Send Notification(notification=w210, notifier=w208, error in (no error)=w206) -> (error out=w209:errorcluster)  [unwired: 1 out]
        n88 = Send Notification(notification=w210, notifier=w211, error in (no error)=w209) -> (error out=w205:errorcluster)  [unwired: 1 out]
      }
      frame "Check if Refnum Update" {
        # "Not used Function"
        n89 = Unbundle By Name(w217) -> ("Initialization.Update Refnums"=w221:bool)
        n90 = case shown="True" w221 {
          tunnel: w218 -> [w226 w231]
          tunnel: [w223 w228] -> w219
          tunnel: w220 -> [w222 w227]
          frame True {
            n91 = Unbundle By Name(w226) -> ("Plot Data"=w224:refnum<queue>)
            n92 = call "Enqueue Message (Single).vi"("error in (no error)"=w222, "Message"="Continue Initialize", "Message Queue"=w224) -> ("error out"=w223:errorcluster)  [unwired: 1 in, 7 out]
          }
          frame False {
            n93 = Unbundle By Name(w231) -> ("Plot Data"=w229:refnum<queue>)
            n94 = call "Enqueue Message (Single).vi"("error in (no error)"=w227, "Message"="Check if Refnum Update", "Message Queue"=w229) -> ("error out"=w228:errorcluster)  [unwired: 1 in, 7 out]
          }
        }
      }
      frame "Continue Initialize" {
        # "Not used Function"
        n95 = Unbundle By Name(w235) -> ("Plot Data"=w232:refnum<queue>)
        n96 = call "Enqueue Message (Single).vi"("error in (no error)"=w234, "Message"="Start Python Session", "Message Queue"=w232) -> ("error out"=w240:errorcluster)  [unwired: 1 in, 7 out]
        n97 = call "Enqueue Message (Single).vi"("error in (no error)"=w240, "Message"="Set Datastructures to Default", "Message Queue"=w232) -> ("error out"=w237:errorcluster)  [unwired: 1 in, 7 out]
        n98 = call "Enqueue Message (Single).vi"("error in (no error)"=w237, "Message"="Ready", "Message Queue"=w232) -> ("error out"=w236:errorcluster)  [unwired: 1 in, 7 out]
      }
    }
    n99 = call "Message Handling Loop.vi"("error in (no error)"=w13, "Message Queue"=w11) -> ("dup error in"=w12:errorcluster)  [unwired: 9 out]
  }
  "error out" <- w3
